vi "NanotecSMCPDDriver.Initialize.vi"(0 "VISA resource name":refnum<visa-resource-name>, 1 "contollerID":i32=-1, 2 "ID Query (True)":bool=TRUE, 3 "Reset (True)":bool=TRUE, 5 "error in (no error)":errorcluster, 8 "Serial Configuration":T1={"Baud Rate"=19200, "Parity"=0, "Data Bits"=8, "Stop Bits"=10, "Flow Control"=0} {"Flow Control" items=["None", "XON/XOFF", "RTS/CTS", "XON/XOFF & RTS/CTS", "DTR/DSR", "XON/XOFF & DTR/DSR"]; "Stop Bits" items=["1.0"=10, "1.5"=15, "2.0"=20]; "Data Bits" items=["7"=7, "8"=8]; "Parity" items=["None", "Odd", "Even", "Mark", "Space"]; "Baud Rate" items=["300"=300, "600"=600, "1200"=1200, "2400"=2400, "4800"=4800, "9600"=9600, "19200"=19200]}) -> (14 "VISA resource name out":refnum<visa-resource-name>, 15 "contollerID out":i32=-1, 19 "error out":errorcluster)   [LabVIEW 2014, in "NanotecSMCPDDriver.lvlib"]
doc: "Establishes communication with the instrument and optionally performs an instrument identification query and/or an instrument reset. It also places the instrument in a default state needed for other instrument driver operations. Therefore, call this VI before calling other instrument driver VIs for this instrument. Generally, you need to call the Initialize VI only once at the beginning of an application."
uses:
  NanotecSMCPDDriver.lvlib
panel:
  # "(c) 2009 GSI.  ALL RIGHTS RESERVED."
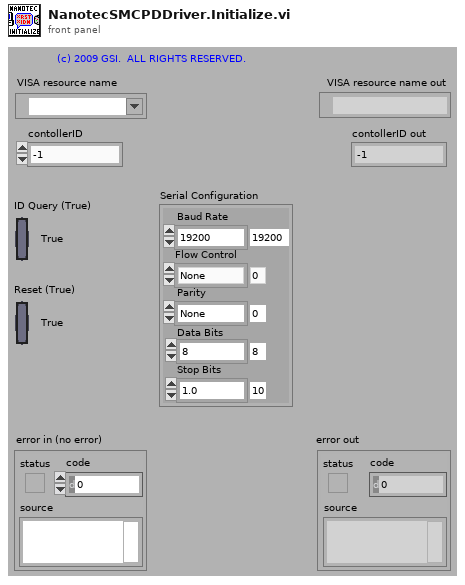
[diagram p1: front panel]
types:
  T1 = cluster{"Baud Rate":u32, "Parity":u16, "Data Bits":u16, "Stop Bits":u16, "Flow Control":u16}
  T2 = enum16{"unknown", "add", "remove", "get", "cleanup"}
  T3 = typedef "NanotecSMCPDDriver.lvlib/NanotecSMCPDDriver.hardware types.ctl" = enum16{"unknown", "PD4", "PD4Ic", "PD2Ic", "SMCI32", "SMCI47"}
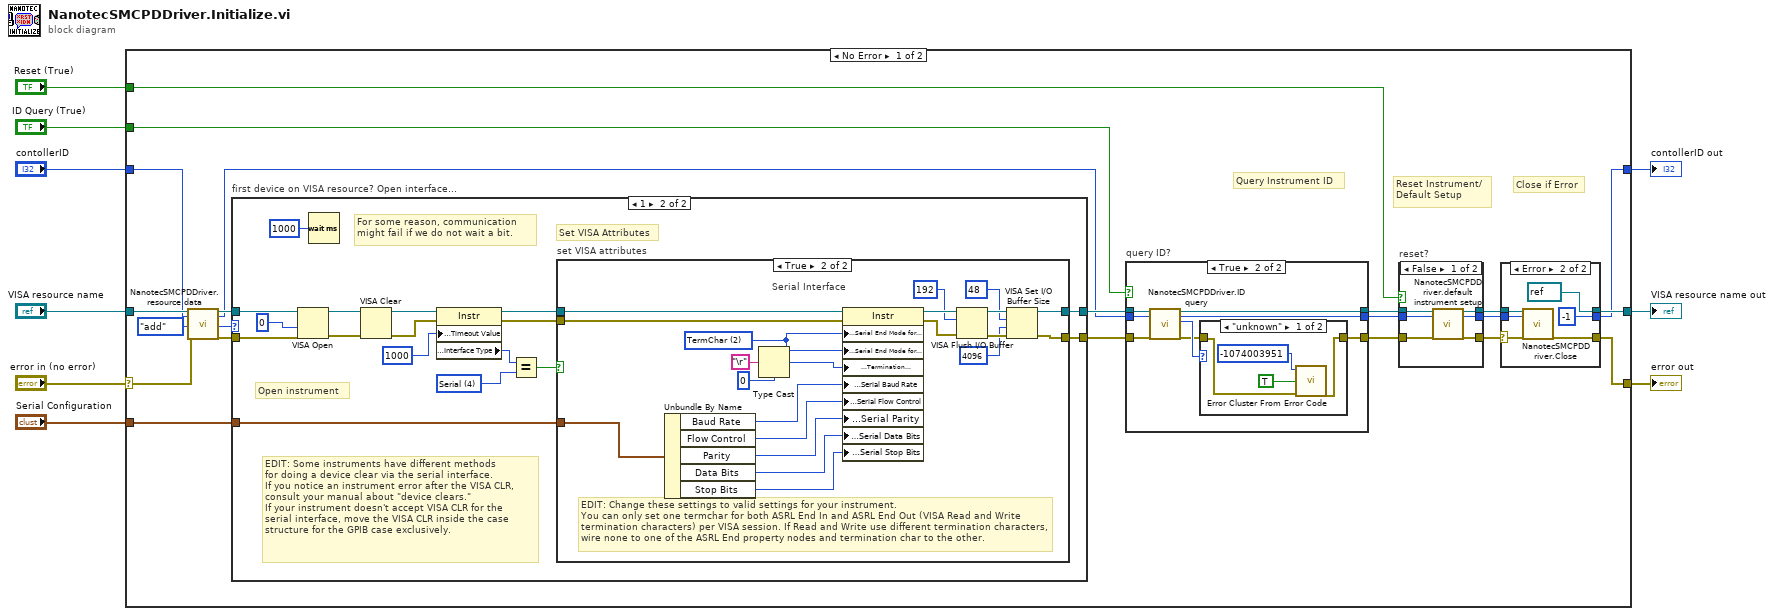
[diagram p0: block diagram]
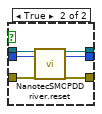
[diagram p5: hidden frame]
diagram:
  n1 = case shown="No Error" "error in (no error)" {
    selector: "error in (no error)" -> [w14 w113]
    tunnel: [w29 w112] -> w9
    tunnel: [w28 w113] -> w8
    tunnel: [w23 w111] -> w7
    tunnel: "VISA resource name" -> [w21 w112]
    tunnel: "contollerID" -> [w18 w111]
    tunnel: "ID Query (True)" -> [w12 _]
    tunnel: "Reset (True)" -> [w11 _]
    tunnel: "Serial Configuration" -> [w10 _]
    frame No Error {
      # "Close if Error"
      # "Query Instrument ID"
      # "Reset Instrument/\nDefault Setup"
      n2 = call "NanotecSMCPDDriver.resource data.vi"("VISAresource"=w21, "contollerID"=w18, "action"=T2."add", "error in (no error)"=w14) -> ("VISAresource out"=w20:refnum<visa-resource-name>, "contollerID out"=w17:i32, "connectionCounter"=w15:i32, "error out"=w19:errorcluster)  [unwired: 11 in, 1 out]
      n3 = case "first device on VISA resource? Open interface..." shown="1" w15 {
        tunnel: [w33 w39] -> w22
        tunnel: w20 -> [w33 w38]
        tunnel: w19 -> [w32 w37]
        tunnel: [w32 w36] -> w16
        tunnel: w10 -> [_ w34]
        frame 0, Default {
        }
        frame 1 {
          w45 = u16 4 items=["GPIB"=1, "VXI"=2, "GPIB-VXI"=3, "Serial"=4, "PXI"=5, "TCPIP"=6, "USB"=7] ("Interface Information:Interface Type")
          # "For some reason, communication\nmight fail if we do not wait a bit."
          # "EDIT: Some instruments have different methods\nfor doing a device clear via the serial interface.  \nIf you notice an instrument error after the VISA CLR,\nconsult your manual about \"device clears.\"  \nIf your instrument doesn't accept VISA CLR for the\nserial interface, move the VISA CLR inside the case \nstructure for the GPIB case exclusively."
          # "Set VISA Attributes"
          # "Open instrument"
          n4 = VISA Open(access mode=u32 0, error in (no error)=w37, VISA resource name=w38) -> (VISA resource name=w43:refnum<visa-resource-name>, error out=w42:errorcluster)  [unwired: 2 in]
          n5 = Wait (ms)(milliseconds to wait=u32 1000) -> ()  [unwired: 1 out]
          n6 = VISA Clear(VISA resource name=w43, error in (no error)=w42) -> (VISA resource name out=w41:refnum<visa-resource-name>, error out=w40:errorcluster)
          n7 = property on="Property Node" class="Instr"(reference=w41, error in=w40, "General Settings:Timeout Value"=u32 1000) -> (reference out=w48:refnum<visa-resource-name>, error out=w47:errorcluster, "Interface Information:Interface Type"=w50:u16)
          n8 = Equal?(x=w50, y=w45) -> (x = y?=w46:bool)
          n9 = case "set VISA attributes" shown="True" w46 {
            tunnel: [w51 w70] -> w39
            tunnel: [w52 w67] -> w36
            tunnel: w48 -> [w51 w72]
            tunnel: w47 -> [w52 w73]
            tunnel: w34 -> [_ w53]
            frame False {
              # "EDIT: Remove interfaces not\nsupported by your instrument."
              # "GPIB, TCP/IP, and USB Interface"
            }
            frame True {
              w60 = u16 2 items=["None", "LastBit", "TermChar"] ("Serial Settings:Serial End Mode for Reads")
              # "EDIT: Change these settings to valid settings for your instrument.\nYou can only set one termchar for both ASRL End In and ASRL End Out (VISA Read and Write termination characters) per VISA session. If Read and Write use different termination characters, wire none to one of the ASRL End property nodes and termination char to the other."
              # "Serial Interface"
              n10 = Unbundle By Name(w53) -> ("Baud Rate"=w58:u32, "Flow Control"=w55:u16, "Parity"=w56:u16, "Data Bits"=w57:u16, "Stop Bits"=w54:u16)
              n11 = Type Cast(type=u8 0, x="\r" ("Carriage Return Constant")) -> (*(type *) &x=w59:u8)
              n12 = property on="Property Node" class="Instr"(reference=w72, error in=w73, "Serial Settings:Serial End Mode for Reads"=w60, "Serial Settings:Serial End Mode for Writes"=w60, "Message Based Settings:Termination Character"=w59, "Serial Settings:Serial Baud Rate"=w58, "Serial Settings:Serial Flow Control"=w55, "Serial Settings:Serial Parity"=w56, "Serial Settings:Serial Data Bits"=w57, "Serial Settings:Serial Stop Bits"=w54) -> (reference out=w66:refnum<visa-resource-name>, error out=w69:errorcluster)
              n13 = VISA Flush I/O Buffer(VISA resource name=w66, mask (16)=u16 192, error in (no error)=w69) -> (VISA resource name out=w71:refnum<visa-resource-name>, error out=w68:errorcluster)
              n14 = VISA Set I/O Buffer Size(VISA resource name=w71, mask (16)=u16 48, size (4096)=u32 4096 ("size (0)"), error in (no error)=w68) -> (VISA resource name out=w70:refnum<visa-resource-name>, error out=w67:errorcluster)
            }
          }
        }
      }
      n15 = case "query ID?" shown="True" w12 {
        tunnel: [w96 w98] -> w30
        tunnel: [w97 w104] -> w31
        tunnel: w22 -> [w97 w105]
        tunnel: w16 -> [w96 w102]
        tunnel: [w95 w103] -> w25
        tunnel: w17 -> [w95 w101]
        frame False {
        }
        frame True {
          n16 = call "NanotecSMCPDDriver.ID query.vi"("VISA resource name"=w105, "contollerID"=w101, "error in (no error)"=w102) -> ("VISA resource name out"=w104:refnum<visa-resource-name>, "contollerID out"=w103:i32, "hardwareType"=w100:T3, "error out"=w99:errorcluster)  [unwired: 12 in, 1 out]
          n17 = case shown="\"unknown\"" w100 {
            tunnel: w99 -> [w106 w110]
            tunnel: [w107 w110] -> w98
            frame "unknown" {
              n18 = call <vilib>:"Error Cluster From Error Code.vi"("show call chain? (False)"=TRUE, "error in (no error)"=w106, "error code (0)"=-1074003951) -> ("error out"=w107:errorcluster)  [unwired: 6 in]
            }
            frame Default {
            }
          }
        }
      }
      n19 = case "reset?" shown="False" w11 {
        tunnel: w30 -> [w87 w94]
        tunnel: [w86 w89] -> w26
        tunnel: w31 -> [w88 w93]
        tunnel: [w85 w91] -> w27
        tunnel: w25 -> [w84 w92]
        tunnel: [w83 w90] -> w24
        frame False {
          n20 = call "NanotecSMCPDDriver.default instrument setup.vi"("VISA resource name"=w88, "contollerID"=w84, "error in (no error)"=w87) -> ("VISA resource name out"=w85:refnum<visa-resource-name>, "contollerID out"=w83:i32, "error out"=w86:errorcluster)  [unwired: 14 in]
        }
        frame True {
          n21 = call "NanotecSMCPDDriver.reset.vi"("VISA resource name"=w93, "contollerID"=w92, "error in (no error)"=w94) -> ("VISA resource name out"=w91:refnum<visa-resource-name>, "contollerID out"=w90:i32, "error out"=w89:errorcluster)  [unwired: 14 in]
        }
      }
      n22 = case shown="Error" w26 {
        selector: w26 -> [w75 w80]
        tunnel: w27 -> [w76 w81]
        tunnel: [w76 refnum<visa-resource-name> refnum ("VISA resource name out")] -> w29
        tunnel: [w75 w82] -> w28
        tunnel: w24 -> [w74 w78]
        tunnel: [w74 -1 ("contollerID out")] -> w23
        frame No Error {
        }
        frame Error {
          n23 = call "NanotecSMCPDDriver.Close.vi"("VISA resource name"=w81, "contollerID"=w78, "error in (no error)"=w80) -> ("error out"=w82:errorcluster)  [unwired: 16 in]
        }
      }
    }
    frame Error {
    }
  }
  "VISA resource name out" <- w9
  "error out" <- w8
  "contollerID out" <- w7
